vi "splitControl.vi"() -> (1 "JoystickDevRef 2":T1, 2 "JoystickDevRef":T1)   [LabVIEW 2016]
uses:
  <vilib>/Rock Robotics/WPI/Joystick/WPI_JoystickDevRef.ctl
  <vilib>/Rock Robotics/WPI/Joystick/WPI_JoystickDeviceEnum.ctl
  <vilib>/Rock Robotics/WPI/Utilities/WPI_GetSetVariantRefNum.vi
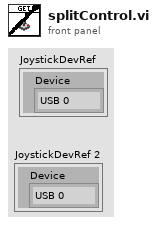
[diagram p1: front panel]
types:
  T1 = typedef "WPI_JoystickDevRef.ctl" = cluster{"Device":T2}
  T2 = typedef "WPI_JoystickDeviceEnum.ctl" = enum16{"USB 0", "USB 1", "USB 2", "USB 3", "USB 4", "USB 5"}
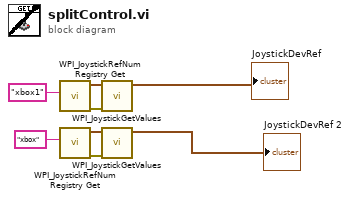
[diagram p0: block diagram]
diagram:
  n1 = call <vilib>:"WPI_JoystickRefNum Registry Get.vi"("refnum name"="xbox1") -> ("error out"=w2:errorcluster, "JoystickDevRef"=w1:T1)  [unwired: 9 in]
  n2 = call <vilib>:"WPI_JoystickRefNum Registry Get.vi"("refnum name"="xbox") -> ("error out"=w5:errorcluster, "JoystickDevRef"=w4:T1)  [unwired: 9 in]
  n3 = call <vilib>:"WPI_JoystickGetValues.vi"("error in (no error)"=w2, "JoystickDevRef"=w1) -> ("JoystickDevRef"=→"JoystickDevRef":T1)  [unwired: 5 in, 4 out]
  n4 = call <vilib>:"WPI_JoystickGetValues.vi"("error in (no error)"=w5, "JoystickDevRef"=w4) -> ("JoystickDevRef"=→"JoystickDevRef 2":T1)  [unwired: 5 in, 4 out]
